vi "destroy.vi"(8 "error in (no error)":errorcluster, 10 "wait_ms":i32, 11 "waitgroup":T1) -> (0 "error out":errorcluster, 3 "unfinished":i32)   [LabVIEW 2015, in "lv-waitgroup.lvlib"]
uses:
  lv-waitgroup.lvlib
  _controls/api_waitgroup.ctl
  private/_controls/waitgroup.ctl
  _controls/data_error.ctl
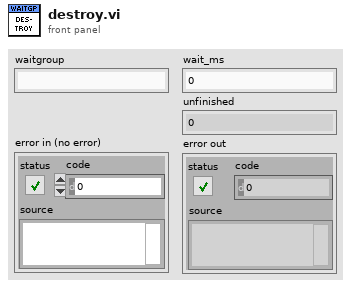
[diagram p1: front panel]
types:
  T1 = typedef "lv-waitgroup.lvlib/api_waitgroup.ctl" = string
  T2 = typedef "lv-waitgroup.lvlib/waitgroup.ctl" = cluster{"waitgroup":refnum<queue>, "queues":variant}
  T3 = typedef "lv-waitgroup.lvlib/data_error.ctl" = enum16{"<data_error>", "unable_to_generate_id", "waitgroup_not_found", "<null>"}
  T4 = typedef "lv-waitgroup.lvlib/references.ctl" = cluster{"waitgroups":refnum<data-value>}
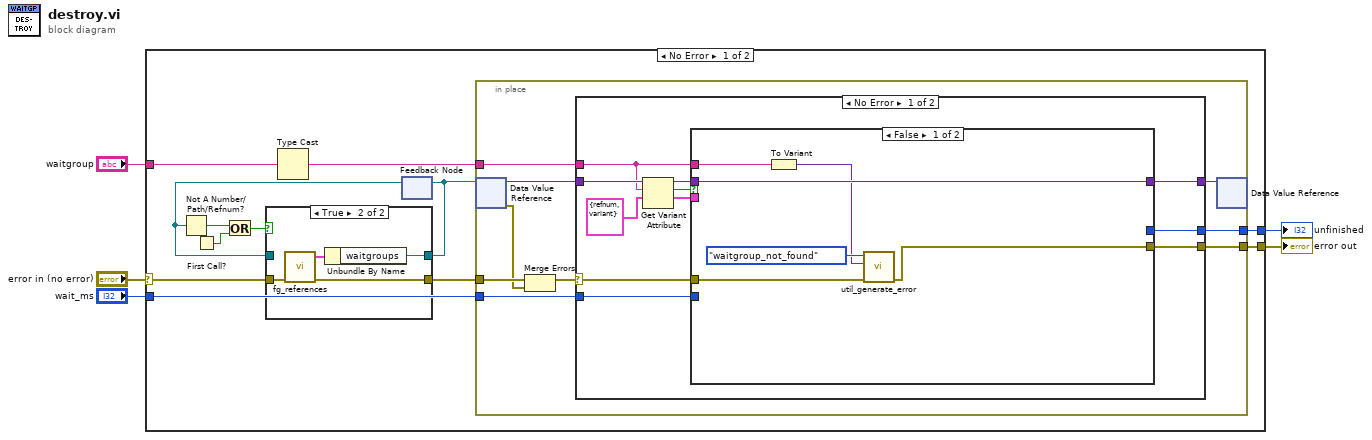
[diagram p0: block diagram]
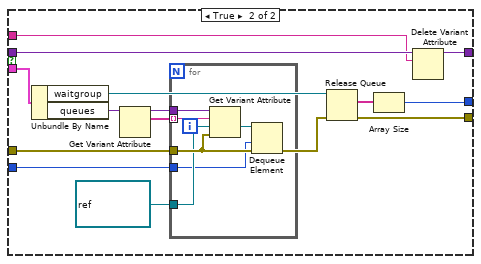
[diagram p3: hidden frame]
diagram:
  n1 = case shown="No Error" "error in (no error)" {
    selector: "error in (no error)" -> [w16 w72]
    tunnel: "waitgroup" -> [w15 _]
    tunnel: [w13 w72] -> w3
    tunnel: [w12 _] -> w2
    tunnel: "wait_ms" -> [w6 _]
    frame No Error {
      n2 = First Call?() -> (First Call?: T/F=w9:bool)
      n3 = Type Cast(x=w15) -> (*(type *) &x=w14:string)  [unwired: 1 in]
      n4 = feedback #1() -> (w8:refnum<data-value>)  [unwired: 1 in]
      n5 = Not A Number/Path/Refnum?(number/path/refnum=w8) -> (NaN/Path/Refnum?=w10:bool)
      n6 = Or(x=w10, y=w9) -> (x .or. y?=w7:bool)
      n7 = case shown="True" w7 {
        tunnel: [w19 w22] -> w17
        tunnel: w16 -> [w19 w21]
        tunnel: [w18 w20] -> w11
        tunnel: w8 -> [w18 _]
        frame False {
        }
        frame True {
          n8 = call "fg_references.vi"("error in (no error)"=w21) -> ("error out"=w22:errorcluster, "references out"=w23:T4)  [unwired: 9 in]
          n9 = Unbundle By Name(w23) -> ("waitgroups"=w20:refnum<data-value>)
        }
      }
      n10 = feedback-in #1(w11) -> ()
      n11 = in-place {
        in-place-border: w17 -> [w32]
        in-place-border: w14 -> [w27]
        in-place-border: [w26] -> w13
        in-place-border: [w25] -> w12
        in-place-border: w6 -> [w24]
        n12 = in-place-dvr #2(w11) -> (w31:variant, w30:errorcluster)
        n13 = Merge Errors(w32, w30) -> (w29:errorcluster)
        n14 = case shown="No Error" w29 {
          selector: w29 -> [w40 w71]
          tunnel: w31 -> [w41 w70]
          tunnel: [w38 w70] -> w28
          tunnel: w27 -> [w37 _]
          tunnel: [w35 w71] -> w26
          tunnel: [w34 _] -> w25
          tunnel: w24 -> [w33 _]
          frame No Error {
            n15 = Get Variant Attribute(Variant=w41, name=w37, default value (empty Variant)=T2 {"waitgroup"=refnum, "queues"=variant(refnum<queue>[] [])} ("shared_data")) -> (duplicate Variant=w39:variant, found=w36:bool, value=w42:T2)  [unwired: 1 in, 1 out]
            n16 = case shown="False" w36 {
              tunnel: w42 -> [_ w63]
              tunnel: w40 -> [w47 w56]
              tunnel: w39 -> [w49 w55]
              tunnel: [w49 w54] -> w38
              tunnel: w37 -> [w45 w53]
              tunnel: [w46 w52] -> w35
              tunnel: [_ w51] -> w34
              tunnel: w33 -> [_ w50]
              frame False {
                n17 = To Variant(anything=w45) -> (Variant=w44:variant)
                n18 = call "util_generate_error.vi"("error in (no error)"=w47, "data"=w44, "data_error"=data_error."waitgroup_not_found") -> ("error out"=w46:errorcluster)  [unwired: 8 in]
              }
              frame True {
                n19 = Unbundle By Name(w63) -> ("waitgroup"=w57:refnum<queue>, "queues"=w61:variant)
                n20 = Get Variant Attribute(Variant=w61) -> (duplicate Variant=w59:variant, names=w60:string[])  [unwired: 3 in, 2 out]
                n21 = for {
                  tunnel: w59 -> [w69]
                  tunnel: w56 -> [w66]
                  tunnel: w60 -> [w68] mode=indexing
                  tunnel: refnum<queue> refnum ("queue") -> [w67]
                  tunnel: w50 -> [w64]
                  n22 = Get Variant Attribute(Variant=w69, name=w68, default value (empty Variant)=w67, error in=w66) -> (value=w65:refnum<queue>)  [unwired: 3 out]
                  n23 = Dequeue Element(queue=w65, timeout in ms (-1)=w64, error in (no error)=w66) -> ()  [unwired: 4 out]
                }
                n24 = Release Queue(queue=w57, error in (no error)=w56) -> (remaining elements=w62:string[], error out=w52:errorcluster)  [unwired: 1 in, 1 out]
                n25 = Array Size(array=w62) -> (size(s)=w51:i32)
                n26 = Delete Variant Attribute(6:w53, 7:w55) -> (3:w54:variant)  [unwired: 1 in, 2 out]
              }
            }
          }
          frame Error {
          }
        }
        n27 = in-place-dvr #2(w28) -> ()  [unwired: 2 out]
      }
    }
    frame Error {
    }
  }
  "error out" <- w3
  "unfinished" <- w2
